vi "Reports_BuildSQLQuery.vi"(8 "error in (no error)":errorcluster, 11 "Array of Event Indexes":string[](array[string])) -> (0 "error out":errorcluster, 2 "SQL Query":string, 3 "Array of Request URLs":string[](array[string]))   [LabVIEW 2014, in "FIRST Reports.lvlib"]
uses:
  FIRST Reports.lvlib
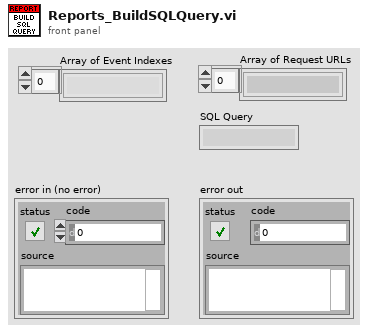
[diagram p1: front panel]
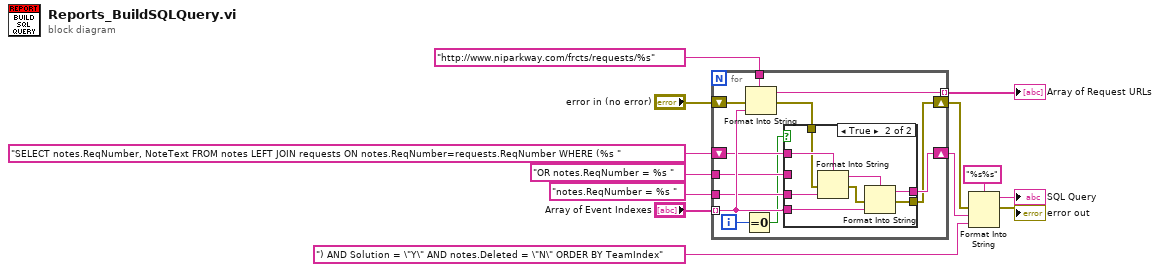
[diagram p0: block diagram]
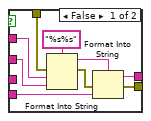
[diagram p2: hidden frame]
diagram:
  n1 = for {
    tunnel: "Array of Event Indexes" -> [w23] mode=indexing
    tunnel: "http://www.niparkway.com/frcts/requests/%s" ("1") -> [w25]
    tunnel: [w24] -> w6 mode=indexing
    tunnel: "notes.ReqNumber = %s " ("4") -> [w22]
    tunnel: "OR notes.ReqNumber = %s " ("3") -> [w19]
    shift-right: [w20] -> w8
    shift-left: "SELECT notes.ReqNumber, NoteText FROM notes LEFT JOIN requests ON notes.ReqNumber=requests.ReqNumber WHERE (%s " ("2") -> [w21]
    shift-right: [w14] -> w12
    shift-left: "error in (no error)" -> [w18]
    i -> [w16]
    n2 = Equal To 0?(x=w16) -> (x = 0?=w15:bool)
    n3 = Format Into String(format string=w25, error in=w18, w23) -> (resulting string=w24:string, error out=w17:errorcluster)  [unwired: 1 in]
    n4 = case shown="True" w15 {
      tunnel: w21 -> [w30 w42]
      tunnel: w22 -> [_ w41]
      tunnel: w23 -> [w33 w39]
      tunnel: [w32 w38] -> w20
      tunnel: w19 -> [w31 _]
      tunnel: w17 -> [w28 w37]
      tunnel: [w26 w35] -> w14
      frame False {
        n5 = Format Into String(format string="%s%s", error in=w28, w30, w31) -> (resulting string=w34:string, error out=w27:errorcluster)  [unwired: 1 in]
        n6 = Format Into String(format string=w34, error in=w27, w33) -> (resulting string=w32:string, error out=w26:errorcluster)  [unwired: 1 in]
      }
      frame True {
        n7 = Format Into String(format string=w42, error in=w37, w41) -> (resulting string=w40:string, error out=w36:errorcluster)  [unwired: 1 in]
        n8 = Format Into String(format string=w40, error in=w36, w39) -> (resulting string=w38:string, error out=w35:errorcluster)  [unwired: 1 in]
      }
    }
  }
  "Array of Request URLs" <- w6
  n9 = Format Into String(format string="%s%s", error in=w12, w8, ") AND Solution = \"Y\" AND notes.Deleted = \"N\" ORDER BY TeamIndex" ("5")) -> (resulting string=→"SQL Query":string, error out=→"error out":errorcluster)  [unwired: 1 in]
